vi "Close Window.vi"(8 "error in (no error)":errorcluster, 11 "HWND":u32) -> (0 "error out":errorcluster)   [LabVIEW 2019, in "LV MDI.lvclass"]
doc: "Close specified window."
uses:
  LV MDI.lvclass
  user32.dll
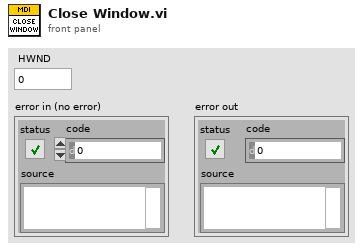
[diagram p1: front panel]
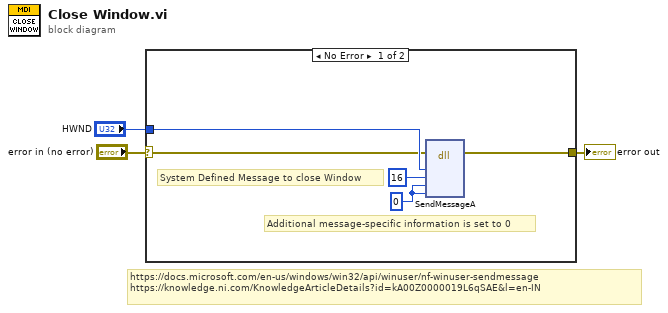
[diagram p0: block diagram]
diagram:
  # "https://docs.microsoft.com/en-us/windows/win32/api/winuser/nf-winuser-sendmessage\nhttps://knowledge.ni.com/KnowledgeArticleDetails?id=kA00Z0000019L6qSAE&l=en-IN"
  n1 = case shown="No Error" "error in (no error)" {
    selector: "error in (no error)" -> [w7 w9]
    tunnel: "HWND" -> [w8 _]
    tunnel: [w6 w9] -> w1
    frame No Error {
      w5 = u32 0 ("wParam")
      # "Additional message-specific information is set to 0"
      # "System Defined Message to close Window"
      n2 = dll-call lib="user32.dll" fn="SendMessageA"(error in=w7, "hwnd"=w8, "msg"=u32 16, "wParam"=w5, "lParam"=w5) -> (error out=w6:errorcluster)  [unwired: 7 in, 1 out]
    }
    frame Error {
    }
  }
  "error out" <- w1
